vi "Initialize Instrument.vi"(8 "error in (no error)":errorcluster, 10 "Instr Resource Str":string, 11 "DSSP.lvclass in":refnum<class "DSSP.lvclass">) -> (0 "error out":errorcluster, 3 "DSSP.lvclass out":refnum<class "DSSP.lvclass">)   [LabVIEW 2010, in "DSSP.lvclass"]
uses:
  DSSP.lvclass
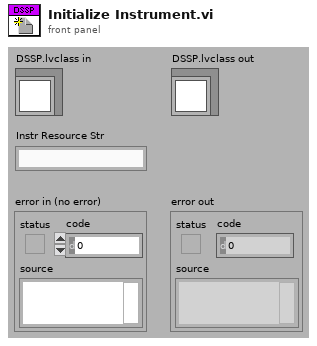
[diagram p1: front panel]
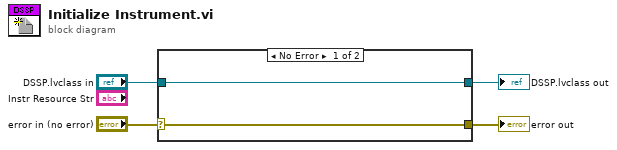
[diagram p0: block diagram]
diagram:
  n1 = case shown="No Error" "error in (no error)" {
    selector: "error in (no error)" -> [w6 w7]
    tunnel: [w6 w7] -> w3
    tunnel: [w5 w8] -> w1
    tunnel: "DSSP.lvclass in" -> [w5 w8]
    frame No Error {
    }
    frame Error {
    }
  }
  "error out" <- w3
  "DSSP.lvclass out" <- w1
